vi "Evaluate tax.vi"(8 "error in (no error)":errorcluster, 10 "Annual ressource":dbl, 11 "Impot in":refnum<class "Impot.lvclass">) -> (0 "error out":errorcluster, 2 "Tax evaluation":dbl, 3 "Impot out":refnum<class "Impot.lvclass">)   [LabVIEW 2023, in "Impot.lvclass"]
uses:
  Impot.lvclass
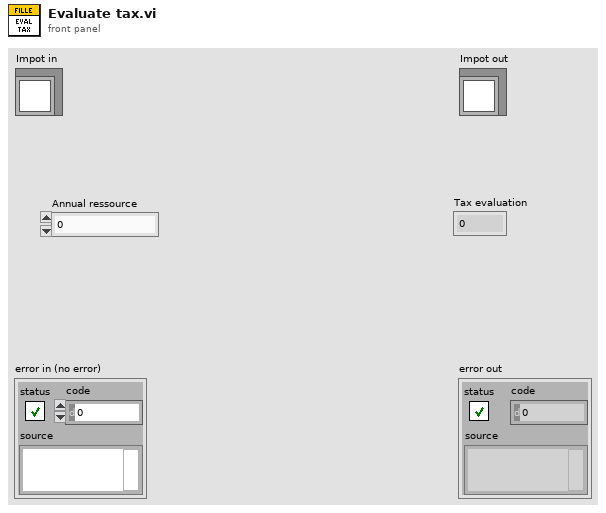
[diagram p1: front panel]
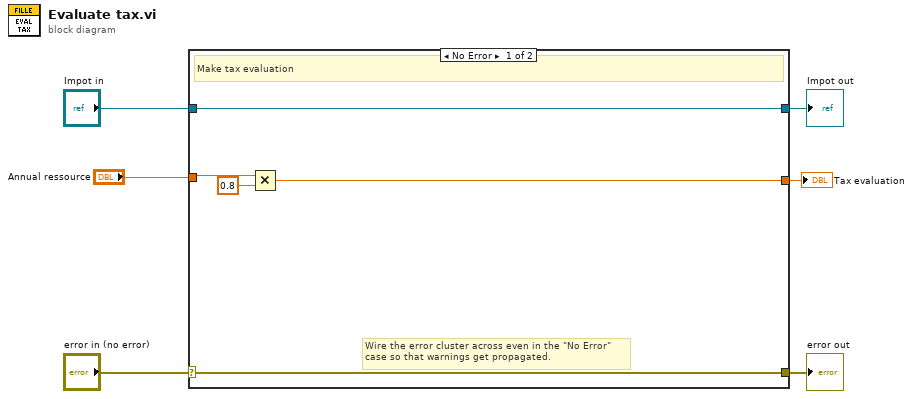
[diagram p0: block diagram]
diagram:
  n1 = case shown="No Error" "error in (no error)" {
    selector: "error in (no error)" -> [w10 w13]
    tunnel: [w10 w13] -> w5
    tunnel: [w11 w12] -> w3
    tunnel: "Impot in" -> [w11 w12]
    tunnel: "Annual ressource" -> [w9 _]
    tunnel: [w7 _] -> w1
    frame No Error {
      # "Wire the error cluster across even in the \"No Error\"\ncase so that warnings get propagated."
      # "Make tax evaluation"
      n2 = Multiply(x=w9, y=0.8) -> (x*y=w7:dbl)
    }
    frame Error {
    }
  }
  "error out" <- w5
  "Impot out" <- w3
  "Tax evaluation" <- w1
